vi "PH_PSDBController.request PSDB writing.vi"(0 "i ref in":refnum<vi>, 2 "Wanted Subsystems":T1[](array[typedef]) items=["Miscellaneous", "fs-Frontend", "ns-Frontend", "PreAmp", "MainAmp", "MAS", "COS", "Beamline", "Experiment Laserbay", "Experiment Laserlabor", "Experiment Z6", "Timing", "Pulsed Power"], 5 "error IO":errorcluster) -> (14 "i ref out":refnum<vi>, 19 "error out":errorcluster)   [LabVIEW 2014, in "PH_PSDBController.lvlib"]
doc: "This VI sets the relevant DIM Service to inform clients to send their data to the PSDB."
uses:
  PH_PSDBController.lvlib
  PH_Basics/PH_PSDBWriter/PH_PSDBWriter.PHELIX-Subsystems.ctl
  CSlibraries-extern/DimLVEvent/LVDimInterface/LVDimInterface.lvlib
  PH_Basics/PH_PSDBWriter/PH_PSDBWriter.lvlib
panel:
  in  "PHELIX Subsystems":T1=2 caption="PHELIX Subsysteme" items=["Miscellaneous", "fs-Frontend", "ns-Frontend", "PreAmp", "MainAmp", "MAS", "COS", "Beamline", "Experiment Laserbay", "Experiment Laserlabor", "Experiment Z6", "Timing", "Pulsed Power"]
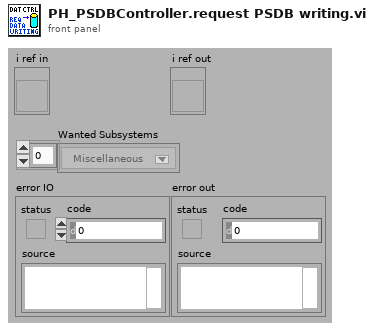
[diagram p1: front panel]
types:
  T1 = typedef "PH_PSDBWriter.lvlib/PH_PSDBWriter.PHELIX-Subsystems.ctl" = i32
  T2 = typedef "PH_PSDBController.lvlib/PH_PSDBController.i attribute.ctl" = cluster{"GUI Refs":cluster{"Data Status":refnum<vi>, "Current Shot ID":refnum<vi>, "active Subsystems":refnum<vi>, "Experiment Description":refnum<vi>, "Shot Comment":refnum<vi>, "Experiment":refnum<vi>, "Shottype":refnum<vi>, "Sequencer SM State":refnum<vi>, "Instances with Errors":refnum<vi>}, "Service ID Shot ID":i32, "Service ID wanted Subsystem":i32, "Data Status":T3, "Shotinformation":cluster{"Current Experiment ID":i32, "Current Shot Type":i32, "Current Comment":string}, "Data taking?":bool, "Service ID current Shottype":i32, "Service ID current Experiment":i32, "Service ID currentShot Comment":i32, "Service ID possible Shottypes":i32, "Service ID possible Experiments":i32, "possible Experiments":T4[], "possible Shottypes":T4[], "List":cluster{"Info":cluster{"Instance":string, "Data Status":T3}[], "GUI Ref":refnum<vi>, "Classname":string}[], "Subsystems Off?":cluster{"PHELIX_Beamline_fs_YLF_BL_Status":bool, "PHELIX_Beamline_ns_BL_Status":bool, "PHELIX_Beamline_PA_Input_BL_Status":bool, "PHELIX_Beamline_PA_MA_BL_Status":bool, "PHELIX_Beamline_MA_Z6_BL_Status":bool, "PHELIX_Beamline_MA_LB_BL_Status":bool, "PHELIX_Beamline_PA_LL_BL_Status":bool}, "PSDB Credentials":T5}
  T3 = typedef "PH_PSDBWriter.lvlib/PH_PSDBWriter.Data Status.ctl" = i16
  T4 = typedef "PSDB.lvlib/PSDB_Info.ctl" = cluster{"Name":string, "Description":string, "ID":i32}
  T5 = typedef "PH_Common.lvlib/PH_Connection.PSDB Credentials.ctl" = cluster{"PW":string, "ID":string, "DS":string}
  T6 = typedef "LVStringsAndValuesArrayTypeDef_I32.ctl" = cluster{"String":string, "Value":i32}[]
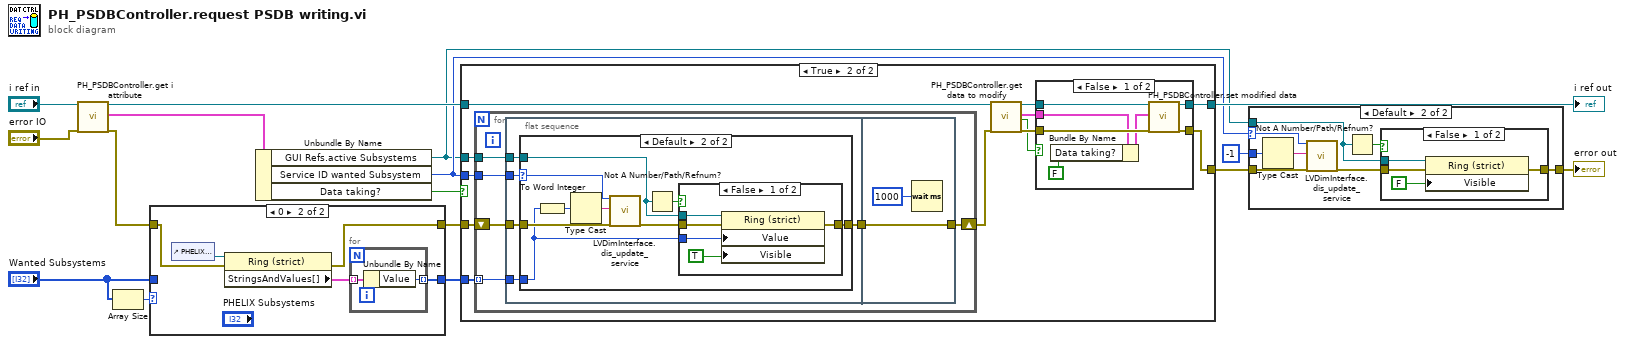
[diagram p0: block diagram]
diagram:
  n1 = call "PH_PSDBController.get i attribute.vi"("i ref in"="i ref in", "error in (no error)"="error IO") -> ("i ref out"=w9:refnum<vi>, "i attribute"=w14:T2, "error out"=w5:errorcluster)  [unwired: 15 in]
  n2 = Array Size(array="Wanted Subsystems") -> (size(s)=w2:i32)
  n3 = case shown="0" w2 {
    tunnel: w5 -> [w17 w23]
    tunnel: [w17 w22] -> w4
    tunnel: [w18 w19] -> w3
    tunnel: "Wanted Subsystems" -> [w18 _]
    frame Default {
    }
    frame 0 {
      n4 = control-ref of="PHELIX Subsystems"() -> (w21:refnum<vi>)
      n5 = property class="Ring (strict)"(reference=w21, error in=w23) -> (error out=w22:errorcluster, "StringsAndValues[]"=w20:T6)  [unwired: 1 out]
      n6 = for {
        tunnel: w20 -> [w25] mode=indexing
        tunnel: [w24] -> w19 mode=indexing
        n7 = Unbundle By Name(w25) -> ("Value"=w24:i32)
      }
    }
  }
  n8 = Unbundle By Name(w14) -> ("GUI Refs.active Subsystems"=w6:refnum<vi>, "Service ID wanted Subsystem"=w7:i32, "Data taking?"=w13:bool)
  n9 = case shown="True" w13 {
    tunnel: [w27 w36] -> w11
    tunnel: w7 -> [_ w39]
    tunnel: w4 -> [w27 w29]
    tunnel: w9 -> [w26 w33]
    tunnel: [w26 w32] -> w8
    tunnel: w6 -> [_ w30]
    tunnel: w3 -> [_ w28]
    frame False {
    }
    frame True {
      n10 = for {
        shift-right: [w53] -> w37
        shift-left: w29 -> [w54]
        tunnel: w39 -> [w51]
        tunnel: w30 -> [w50]
        tunnel: w28 -> [w49] mode=indexing
        n11 = flat-sequence {
          tunnel: w54 -> [w59]
          tunnel: w49 -> [w55]
          tunnel: [w58] -> w52
          tunnel: w51 -> [w57]
          tunnel: w50 -> [w56]
          tunnel: [w77] -> w53
          tunnel: w52 -> [w77]
          frame #0 {
            n12 = case shown="Default" w57 {
              selector: w57 -> [_ w68]
              tunnel: [w60 w65] -> w58
              tunnel: w59 -> [w60 w69]
              tunnel: w55 -> [_ w63]
              tunnel: w56 -> [_ w62]
              frame -1 {
              }
              frame Default {
                n13 = To Word Integer(number=w63) -> (16bit integer=w64:i16)
                n14 = Type Cast(x=w64) -> (*(type *) &x=w67:string)  [unwired: 1 in]
                n15 = call "LVDimInterface.dis_update_service.vi"("my_serviceID"=w68, "data"=w67, "error in (no error)"=w69) -> ("error out"=w66:errorcluster)  [unwired: 14 in, 2 out]
                n16 = Not A Number/Path/Refnum?(number/path/refnum=w62) -> (NaN/Path/Refnum?=w61:bool)
                n17 = case shown="False" w61 {
                  tunnel: w66 -> [w74 w75]
                  tunnel: [w73 w75] -> w65
                  tunnel: w62 -> [w72 _]
                  tunnel: w63 -> [w71 _]
                  frame False {
                    n18 = property class="Ring (strict)"(reference=w72, error in=w74, "Value"=w71, "Visible"=TRUE) -> (error out=w73:errorcluster)  [unwired: 1 out]
                  }
                  frame True {
                  }
                }
              }
            }
          }
          frame #1 {
            n19 = Wait (ms)(milliseconds to wait=u32 1000) -> ()  [unwired: 1 out]
          }
        }
      }
      n20 = call "PH_PSDBController.get data to modify.vi"("i ref in"=w33, "error in (no error)"=w37) -> ("i ref out"=w35:refnum<vi>, "i attribute"=w34:T2, "timed out"=w31:bool, "error out"=w38:errorcluster)  [unwired: 14 in]
      n21 = case shown="False" w31 {
        tunnel: w38 -> [w46 w47]
        tunnel: [w45 w47] -> w36
        tunnel: w35 -> [w44 w48]
        tunnel: w34 -> [w43 _]
        tunnel: [w40 w48] -> w32
        frame False {
          n22 = Bundle By Name(cluster=w43, "Data taking?"=FALSE) -> (w41:T2)
          n23 = call "PH_PSDBController.set modified data.vi"("i ref in"=w44, "i attribute"=w41, "error in (no error)"=w46) -> ("i ref out"=w40:refnum<vi>, "error out"=w45:errorcluster)  [unwired: 15 in]
        }
        frame True {
        }
      }
    }
  }
  "i ref out" <- w8
  n24 = case shown="Default" w7 {
    selector: w7 -> [_ w85]
    tunnel: [w78 w81] -> w10
    tunnel: w11 -> [w78 w86]
    tunnel: i16 -1 -> [_ w83]
    tunnel: w6 -> [_ w80]
    frame -1 {
    }
    frame Default {
      n25 = Type Cast(x=w83) -> (*(type *) &x=w84:string)  [unwired: 1 in]
      n26 = call "LVDimInterface.dis_update_service.vi"("my_serviceID"=w85, "data"=w84, "error in (no error)"=w86) -> ("error out"=w82:errorcluster)  [unwired: 14 in, 2 out]
      n27 = Not A Number/Path/Refnum?(number/path/refnum=w80) -> (NaN/Path/Refnum?=w79:bool)
      n28 = case shown="False" w79 {
        tunnel: w82 -> [w90 w91]
        tunnel: [w89 w91] -> w81
        tunnel: w80 -> [w88 _]
        frame False {
          n29 = property class="Ring (strict)"(reference=w88, error in=w90, "Visible"=FALSE) -> (error out=w89:errorcluster)  [unwired: 1 out]
        }
        frame True {
        }
      }
    }
  }
  "error out" <- w10
